vi "Reply Msg.vi"(8 "error in":errorcluster, 10 "Input":variant, 11 "Target Reply Time Test Actor in":refnum<class "Target Reply Time Test Actor.lvclass">) -> (0 "error out":errorcluster, 2 "Output":variant, 3 "Target Reply Time Test Actor out":refnum<class "Target Reply Time Test Actor.lvclass">)   [LabVIEW 2023, in "Target Reply Time Test Actor.lvlib" / "Target Reply Time Test Actor.lvclass"]
uses:
  Target Reply Time Test Actor.lvclass
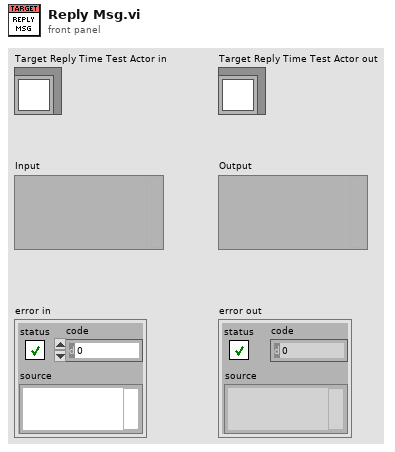
[diagram p1: front panel]
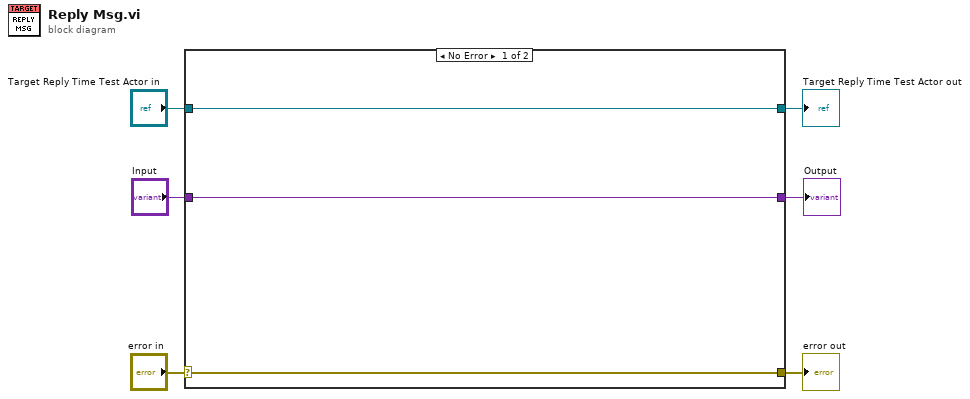
[diagram p0: block diagram]
diagram:
  n1 = case shown="No Error" "error in" {
    selector: "error in" -> [w8 w11]
    tunnel: [w8 w11] -> w5
    tunnel: [w9 w10] -> w3
    tunnel: "Target Reply Time Test Actor in" -> [w9 w10]
    tunnel: "Input" -> [w7 _]
    tunnel: [w7 _] -> w1
    frame No Error {
    }
    frame Error {
    }
  }
  "error out" <- w5
  "Target Reply Time Test Actor out" <- w3
  "Output" <- w1
